vi "RichToFlatnixnet_grpc_ReadStateResponse.vi"(5 "OutputClusterType":T1, 11 "InputCluster":T15) -> (3 "OutputCluster":T1)   [LabVIEW 2025, in "xnet-grpc_client.lvlib"]
uses:
  nixnet_grpc_ReadStateResponse.ctl
  nixnet_grpc_ReadStateValue_value/nixnet_grpc_ReadStateValue_value.lvclass
  nixnet_grpc_ReadStateValue.ctl
  nixnet_grpc_ReadStateResponse_Flat.ctl
  nixnet_grpc_ReadStateValue_Flat.ctl
  nixnet_grpc_CanCommResponse_Flat.ctl
  nixnet_grpc_CanCommState.ctl
  nixnet_grpc_CanLastErr.ctl
  nixnet_grpc_FlexRayCommResponse_Flat.ctl
  nixnet_grpc_FlexRayPocState.ctl
  nixnet_grpc_FlexRayStats_Flat.ctl
  nixnet_grpc_LinCommResponse_Flat.ctl
  nixnet_grpc_LinCommState.ctl
  nixnet_grpc_SessionInfoResponse_Flat.ctl
  nixnet_grpc_SessionInfoState.ctl
  nixnet_grpc_J1939CommState_Flat.ctl
  nixnet_grpc_TimeLocalNetwork_Flat.ctl
  xnet-grpc_client.lvlib
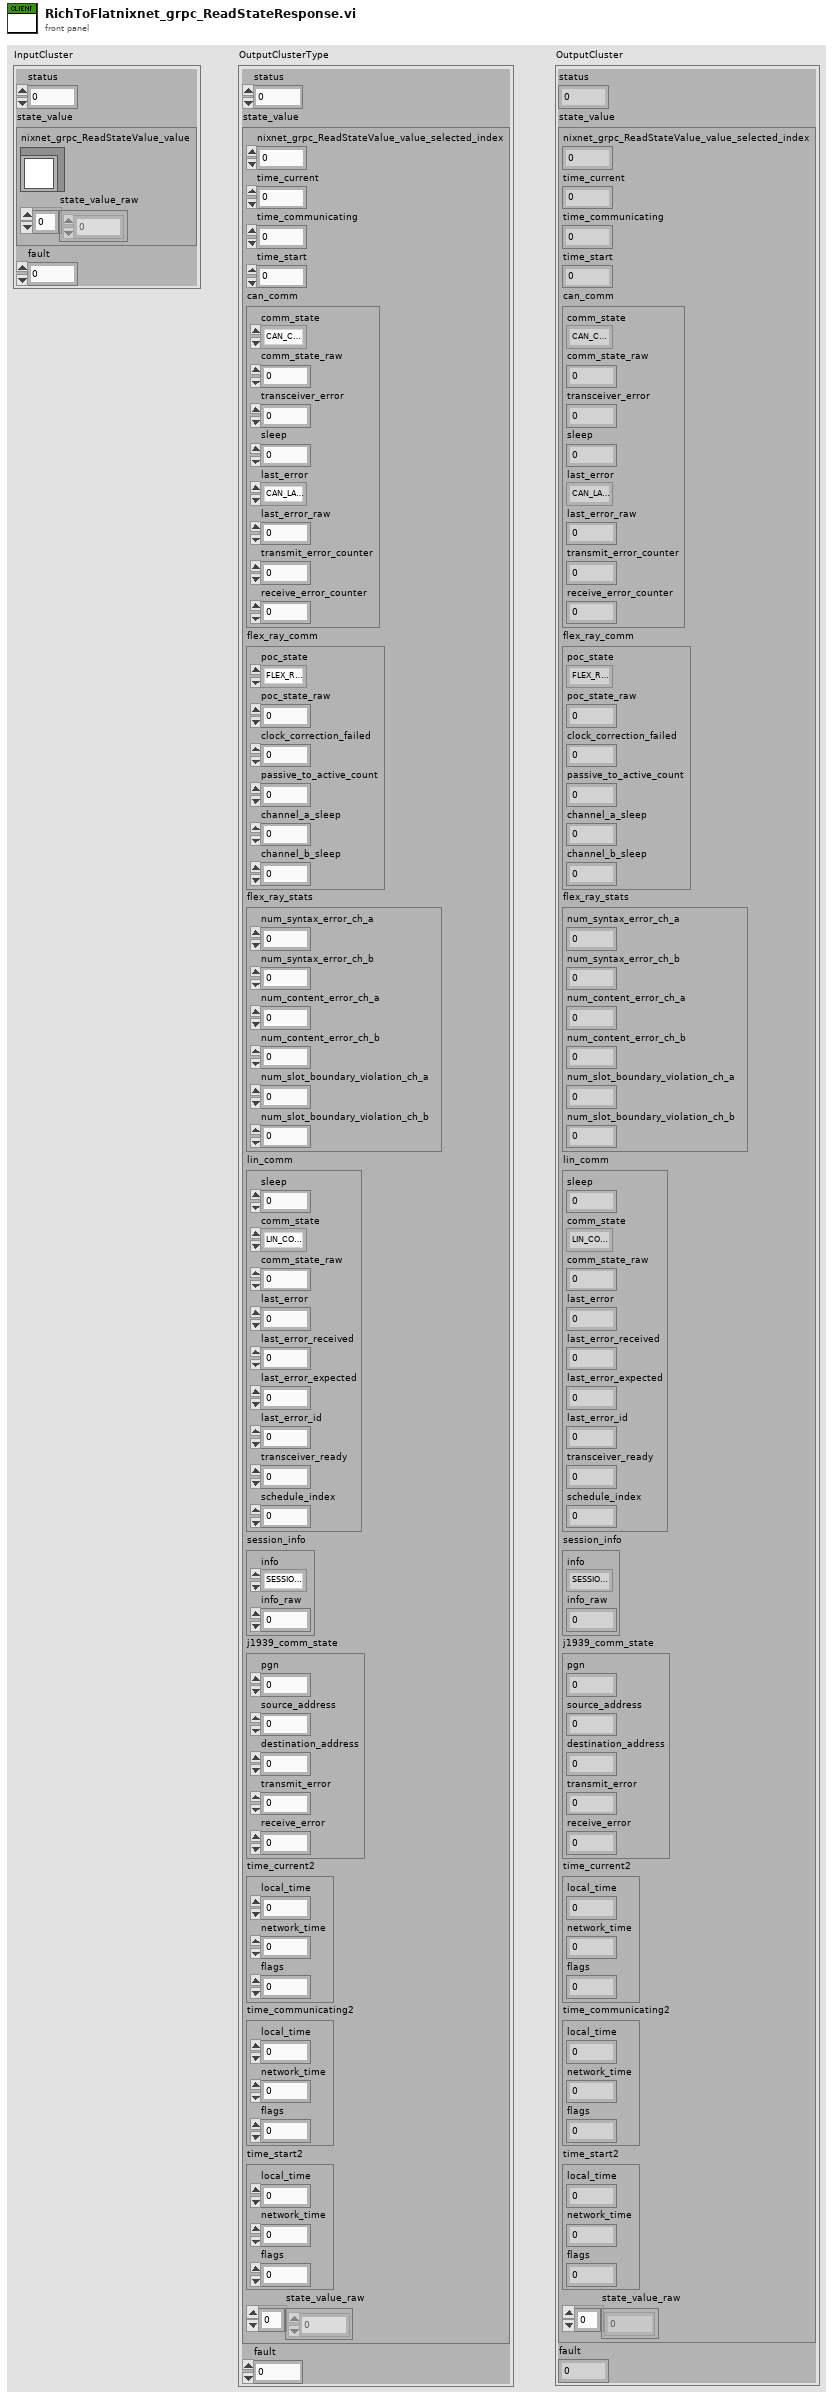
[diagram p1: front panel]
types:
  T1 = typedef "xnet-grpc_client.lvlib/nixnet_grpc_ReadStateResponse_Flat.ctl" = cluster{"status":i32, "state_value":T2, "fault":i32}
  T2 = typedef "xnet-grpc_client.lvlib/nixnet_grpc_ReadStateValue_Flat.ctl" = cluster{"nixnet_grpc_ReadStateValue_value_selected_index":i32, "time_current":u64, "time_communicating":u64, "time_start":u64, "can_comm":T3, "flex_ray_comm":T6, "flex_ray_stats":T8, "lin_comm":T9, "session_info":T11, "j1939_comm_state":T13, "time_current2":T14, "time_communicating2":T14, "time_start2":T14, "state_value_raw":u8[]}
  T3 = typedef "xnet-grpc_client.lvlib/nixnet_grpc_CanCommResponse_Flat.ctl" = cluster{"comm_state":T4, "comm_state_raw":u32, "transceiver_error":u32, "sleep":u32, "last_error":T5, "last_error_raw":u32, "transmit_error_counter":u32, "receive_error_counter":u32}
  T4 = typedef "xnet-grpc_client.lvlib/nixnet_grpc_CanCommState.ctl" = enum32{"CAN_COMM_STATE_ERROR_ACTIVE", "CAN_COMM_STATE_ERROR_PASSIVE", "CAN_COMM_STATE_BUS_OFF", "CAN_COMM_STATE_INIT"}
  T5 = typedef "xnet-grpc_client.lvlib/nixnet_grpc_CanLastErr.ctl" = enum32{"CAN_LAST_ERR_NONE", "CAN_LAST_ERR_STUFF", "CAN_LAST_ERR_FORM", "CAN_LAST_ERR_ACK", "CAN_LAST_ERR_BIT_1", "CAN_LAST_ERR_BIT_0", "CAN_LAST_ERR_CRC"}
  T6 = typedef "xnet-grpc_client.lvlib/nixnet_grpc_FlexRayCommResponse_Flat.ctl" = cluster{"poc_state":T7, "poc_state_raw":u32, "clock_correction_failed":u32, "passive_to_active_count":u32, "channel_a_sleep":u32, "channel_b_sleep":u32}
  T7 = typedef "xnet-grpc_client.lvlib/nixnet_grpc_FlexRayPocState.ctl" = enum32{"FLEX_RAY_POC_STATE_DEFAULT_CONFIG", "FLEX_RAY_POC_STATE_READY", "FLEX_RAY_POC_STATE_NORMAL_ACTIVE", "FLEX_RAY_POC_STATE_NORMAL_PASSIVE", "FLEX_RAY_POC_STATE_HALT", "FLEX_RAY_POC_STATE_MONITOR", "FLEX_RAY_POC_STATE_CONFIG"}
  T8 = typedef "xnet-grpc_client.lvlib/nixnet_grpc_FlexRayStats_Flat.ctl" = cluster{"num_syntax_error_ch_a":u32, "num_syntax_error_ch_b":u32, "num_content_error_ch_a":u32, "num_content_error_ch_b":u32, "num_slot_boundary_violation_ch_a":u32, "num_slot_boundary_violation_ch_b":u32}
  T9 = typedef "xnet-grpc_client.lvlib/nixnet_grpc_LinCommResponse_Flat.ctl" = cluster{"sleep":u32, "comm_state":T10, "comm_state_raw":u32, "last_error":u32, "last_error_received":u32, "last_error_expected":u32, "last_error_id":u32, "transceiver_ready":u32, "schedule_index":u32}
  T10 = typedef "xnet-grpc_client.lvlib/nixnet_grpc_LinCommState.ctl" = enum32{"LIN_COMM_STATE_IDLE", "LIN_COMM_STATE_ACTIVE", "LIN_COMM_STATE_INACTIVE"}
  T11 = typedef "xnet-grpc_client.lvlib/nixnet_grpc_SessionInfoResponse_Flat.ctl" = cluster{"info":T12, "info_raw":u32}
  T12 = typedef "xnet-grpc_client.lvlib/nixnet_grpc_SessionInfoState.ctl" = enum32{"SESSION_INFO_STATE_STOPPED", "SESSION_INFO_STATE_STARTED", "SESSION_INFO_STATE_MIX"}
  T13 = typedef "xnet-grpc_client.lvlib/nixnet_grpc_J1939CommState_Flat.ctl" = cluster{"pgn":u32, "source_address":u32, "destination_address":u32, "transmit_error":u32, "receive_error":u32}
  T14 = typedef "xnet-grpc_client.lvlib/nixnet_grpc_TimeLocalNetwork_Flat.ctl" = cluster{"local_time":u64, "network_time":u64, "flags":u32}
  T15 = typedef "xnet-grpc_client.lvlib/nixnet_grpc_ReadStateResponse.ctl" = cluster{"status":i32, "state_value":T16, "fault":i32}
  T16 = typedef "xnet-grpc_client.lvlib/nixnet_grpc_ReadStateValue.ctl" = cluster{"nixnet_grpc_ReadStateValue_value":refnum<class "nixnet_grpc_ReadStateValue_value.lvclass">, "state_value_raw":u8[]}
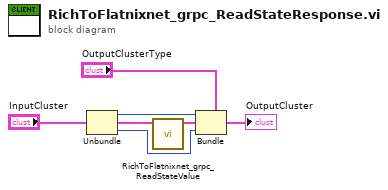
[diagram p0: block diagram]
diagram:
  n1 = Unbundle "Unbundle"("InputCluster") -> ("status"=w4:i32, "state_value"=w3:T16, "fault"=w1:i32)
  n2 = call "RichToFlatnixnet_grpc_ReadStateValue.vi"("InputCluster"=w3) -> ("OutputCluster"=w2:T2)  [unwired: 10 in]
  n3 = Bundle "Bundle"(cluster="OutputClusterType", "status"=w4, "state_value"=w2, "fault"=w1) -> (→"OutputCluster":T1)
